vi "Generate TL and RT.vi"() -> (0 "tl + rt":string)   [LabVIEW 2024, in "OptoMMP.lvlib"]
doc: "Generates a transaction label and retry code for an OptoMMP packet, formatted as a single-byte hexadecimal string. \n\nThis subVI is non-reentrant to ensure that adjacent OptoMMP requests do not have the same transaction ID. \n\nLast updated: 10/8/2025"
uses:
  <instrlib>/OptoMMP/OptoMMP.lvlib
panel:
  # "Copyright (c) 2025 California Institute of Technology (Caltech).\nU.S. Government sponsorship acknowledged.\n\nLicensed under the Apache License, Version 2.0 (the \"License\");\nyou may not use this file except in compliance with the License.\nYou may obtain a copy of the License at\n\n    http://www.apache.org/licenses/LICENSE-2.0\n\nUnless required by applicable law or agreed to in writing, software\ndistributed under the License is distributed on an \"AS IS\" BASIS,\nWITHOUT WARRANTIES OR CONDITIONS OF ANY KIND, either express or implied.\nSee the License for the specific language governing permissions and\nlimitations under the License."
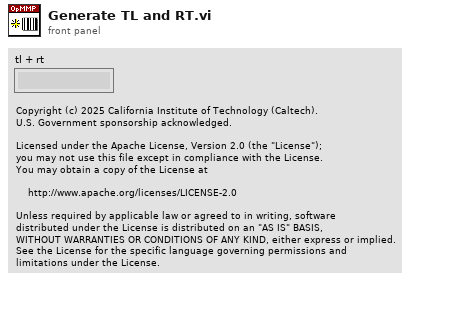
[diagram p1: front panel]
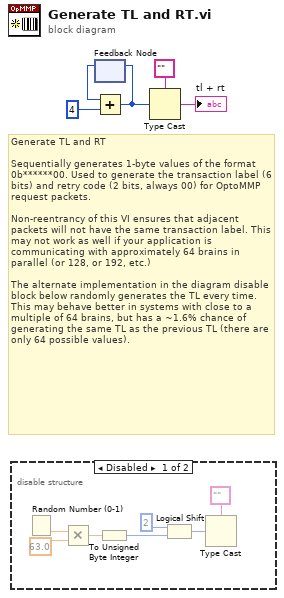
[diagram p0: block diagram]
diagram:
  # "Generate TL and RT\n\nSequentially generates 1-byte values of the format 0b******00. Used to generate the transaction label (6 bits) and retry code (2 bits, always 00) for OptoMMP request packets. \n\nNon-reentrancy of this VI ensures that adjacent packets will not have the same transaction label. This may not work as well if your application is communicating with approximately 64 brains in parallel (or 128, or 192, etc.)\n\nThe alternate implementation in the diagram disable block below randomly generates the TL every time. This may behave better in systems with close to a multiple of 64 brains, but has a ~1.6% chance of generating the same TL as the previous TL (there are only 64 possible values)."
  n1 = disable-structure shown="Disabled" {
    frame Disabled {
      n2 = Random Number (0-1)() -> (number: 0 to 1=w11:dbl)
      n3 = Multiply(x=w11, y=63.0) -> (x*y=w10:dbl)
      n4 = To Unsigned Byte Integer(number=w10) -> (unsigned 8bit integer=w9:u8)
      n5 = Logical Shift(y=i16 2, x=w9) -> (x << y=w6:u8)
      n6 = Type Cast(type="", x=w6) -> ()  [unwired: 1 out]
    }
    frame Enabled {
    }
  }
  n7 = feedback #1() -> (w5:u8)  [unwired: 1 in]
  n8 = Add(x=w5, y=u8 4) -> (x+y=w1:u8)
  n9 = feedback-in #1(w1) -> ()
  n10 = Type Cast(type="", x=w1) -> (*(type *) &x=→"tl + rt":string)
